vi "CloseInterface.vi"(8 "error in (no error)":errorcluster, 9 "handle":i64) -> (0 "error out":errorcluster, 2 "return type":i32)   [LabVIEW 2013, in "MvCameraControl.lvlib"]
doc: "MV_CAMCTRL_API int __stdcall MV_CC_CloseInterface(IN void* handle);"
uses:
  MvCameraControl.lvlib
  MvCameraControl.dll
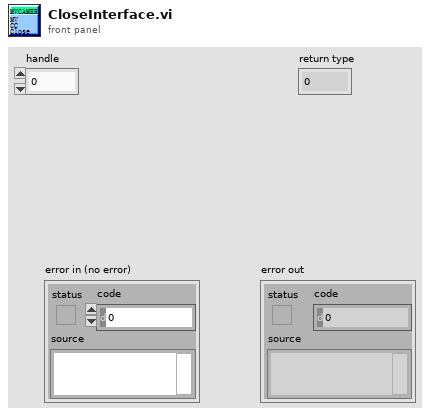
[diagram p1: front panel]
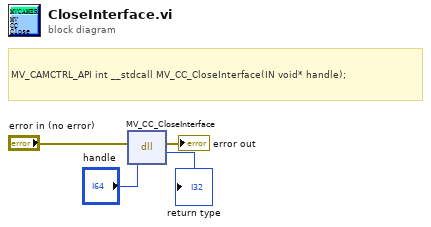
[diagram p0: block diagram]
diagram:
  # "MV_CAMCTRL_API int __stdcall MV_CC_CloseInterface(IN void* handle);"
  n1 = dll-call lib="MvCameraControl.*" fn="MV_CC_CloseInterface"(error in="error in (no error)", "handle"="handle") -> (error out=→"error out":errorcluster, "return type"=→"return type":i32)  [unwired: 3 in, 1 out]
